vi "run.vi"() -> ()   [LabVIEW 2011, in "Hardware.lvlib" / "frequencyCounters.lvlib" / "frequencyCounterController.lvclass"]
uses:
  frequencyCounterController.lvclass
  frequencyCounterController.lvclass/frequencyCounterController.ctl
  BK1823ACounter/BK1823ACounter.lvclass
  FrequencyViewer/FrequencyViewer.lvclass
panel:
  in  "stop":bool
  in  "frequencyController.lvclass":refnum<class "frequencyCounterController.lvclass">
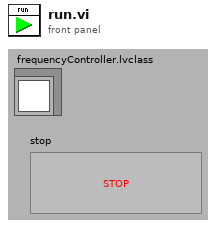
[diagram p1: front panel]
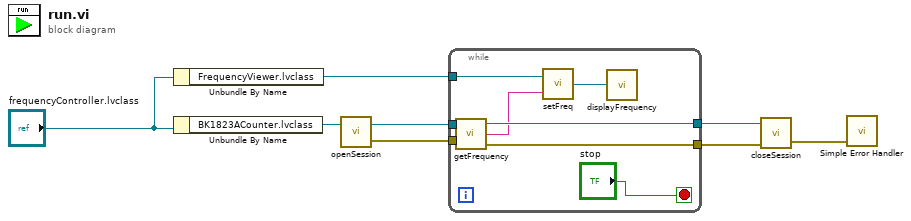
[diagram p0: block diagram]
diagram:
  n1 = Unbundle By Name("frequencyController.lvclass") -> ("FrequencyViewer.lvclass"=w6:refnum<class "FrequencyViewer.lvclass">)
  n2 = Unbundle By Name("frequencyController.lvclass") -> ("BK1823ACounter.lvclass"=w8:refnum<class "BK1823ACounter.lvclass">)
  n3 = call-dynamic "openSession.vi"("BK1823ACounter.lvclass"=w8) -> ("error out"=w4:errorcluster, "BK1823ACounter.lvclass 2"=w5:refnum<class "BK1823ACounter.lvclass">)  [unwired: 1 in]
  n4 = while {
    tunnel: w6 -> [w16]
    tunnel: w5 -> [w15]
    tunnel: w4 -> [w14]
    tunnel: [w13] -> w3
    tunnel: [w12] -> w2
    stop <- "stop" stop-if-true
    n5 = call-dynamic "getFrequency.vi"("BK1823ACounter.lvclass"=w15, "error in (no error)"=w14) -> ("BK1823ACounter.lvclass 2"=w13:refnum<class "BK1823ACounter.lvclass">, "Frequency"=w11:string, "error out"=w12:errorcluster)
    n6 = call "setFreq.vi"("new frequency"=w11, "FrequencyViewer.lvclass"=w16) -> ("FrequencyViewer.lvclass 2"=w10:refnum<class "FrequencyViewer.lvclass">)
    n7 = call "displayFrequency.vi"("FrequencyViewer.lvclass"=w10) -> ()  [unwired: 2 out]
  }
  n8 = call-dynamic "closeSession.vi"("error in (no error)"=w2, "BK1823ACounter.lvclass"=w3) -> ("error out"=w1:errorcluster)  [unwired: 1 out]
  n9 = call <vilib>:"Simple Error Handler.vi"("error in (no error)"=w1) -> ()  [unwired: 4 in, 5 out]
